vi "ClearSpectrum.vi"(8 "error in":errorcluster, 11 "connection ID in":refnum<k5>) -> (0 "error out":errorcluster, 1 "Error Info":T1, 2 "OK":bool, 3 "connection ID out":refnum<k5>, 4 "Log String":string)   [LabVIEW 2020, in "ProdigyRemoteControl.lvlib"]
uses:
  ProdigyRemoteControl.lvlib
  DEFINITIONS/DEF_RcError.ctl
  DEFINITIONS/DEF_RcCmd.ctl
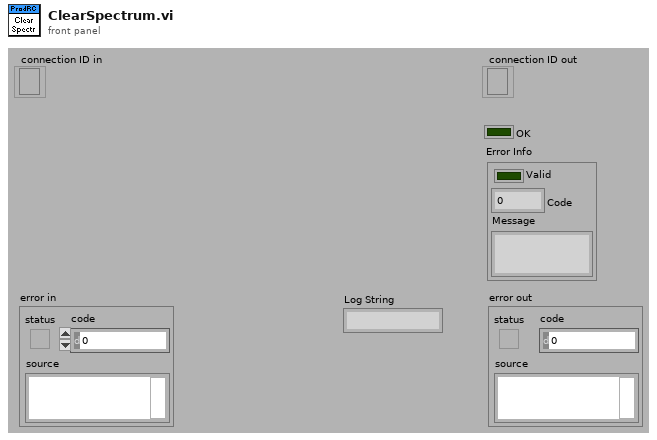
[diagram p1: front panel]
types:
  T1 = typedef "ProdigyRemoteControl.lvlib/DEF_RcError.ctl" = cluster{"Valid":bool, "Code":u16, "Message":string}
  T2 = typedef "ProdigyRemoteControl.lvlib/DEF_RcCmd.ctl" = string
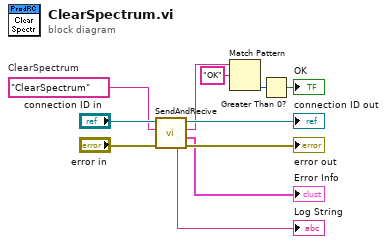
[diagram p0: block diagram]
diagram:
  w7 = T2 "ClearSpectrum"  # ClearSpectrum
  n1 = call "SendAndRecive.vi"("error in"="error in", "Command"=w7, "connection ID in"="connection ID in") -> ("error out"=→"error out":errorcluster, "Error Info"=→"Error Info":T1, "Answer"=w4:string, "connection ID out"=→"connection ID out":refnum<k5>, "Log String"=→"Log String":string)  [unwired: 4 in]
  n2 = Match Pattern(string=w4, regular expression="OK") -> (offset past match=w2:i32)  [unwired: 1 in, 3 out]
  n3 = Greater Than 0?(x=w2) -> (x > 0?=→"OK":bool)
